vi "Set Switch Heater.vi"(1 "error in":T2, 2 "Switch Heater Control":bool, 3 "Communications Config":T1={"GPIB address"=22, "GPIB bus"=0, "connection ID"=refnum, "IP"="192.168.2.200", "Active Comm Interface"=0, "Serial Port"="", "Programmer Type"=0} {"Programmer Type" items=["Model 430", "Model 420"]; "Active Comm Interface" items=["TCP/IP (Model 430 Only)", "RS232", "IEEE488"]}) -> (0 "error out":T2)   [LabVIEW 2018]
panel:
  in  "GPIB Address":cluster{"GPIB address":i16, "GPIB bus":i16}={"GPIB address"=22, "GPIB bus"=0}
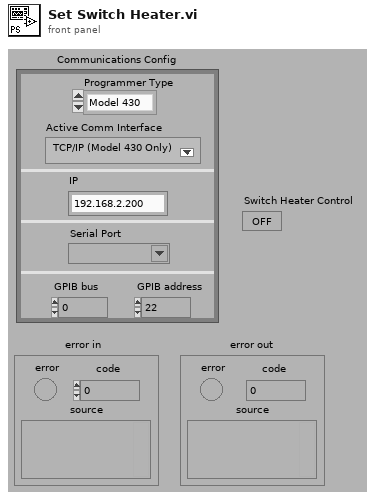
[diagram p1: front panel]
types:
  T1 = cluster{"GPIB address":i16, "GPIB bus":i16, "connection ID":refnum<k5>, "IP":string, "Active Comm Interface":u16, "Serial Port":refnum<visa-resource-name>, "Programmer Type":u16}
  T2 = cluster{"error":bool, "code":i32, "source":string}
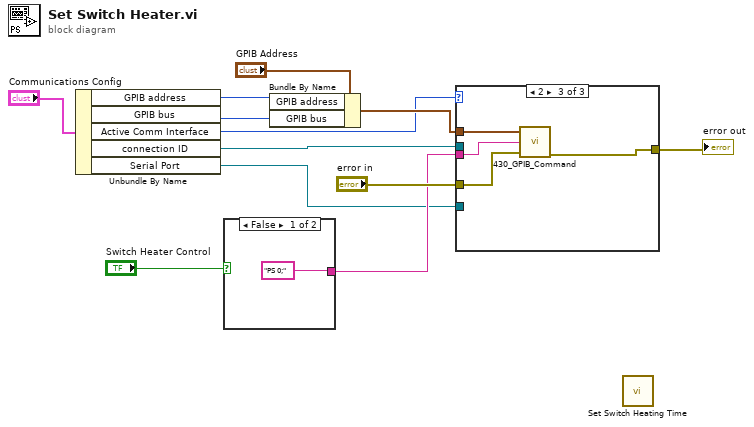
[diagram p0: block diagram]
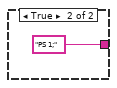
[diagram p2: hidden frame]
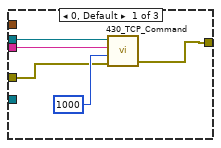
[diagram p3: hidden frame]
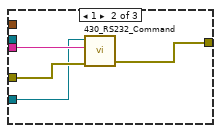
[diagram p4: hidden frame]
diagram:
  n1 = Unbundle By Name("Communications Config") -> ("GPIB address"=w6:i16, "GPIB bus"=w5:i16, "Active Comm Interface"=w4:u16, "connection ID"=w3:refnum<k5>, "Serial Port"=w2:refnum<visa-resource-name>)
  n2 = case shown="False" "Switch Heater Control" {
    tunnel: ["PS 0;" "PS 1;"] -> w8
    frame False {
    }
    frame True {
    }
  }
  n3 = Bundle By Name(cluster="GPIB Address", "GPIB address"=w6, "GPIB bus"=w5) -> (w7:cluster{"GPIB address":i16, "GPIB bus":i16})
  n4 = case shown="2" w4 {
    tunnel: w7 -> [_ _ w24]
    tunnel: "error in" -> [w18 w22 w27]
    tunnel: [w15 w21 w26] -> w11
    tunnel: w8 -> [w17 w23 w25]
    tunnel: w3 -> [w16 _ _]
    tunnel: w2 -> [_ w20 _]
    frame 0, Default {
      n5 = call "430_TCP_Command.vi"("error in (no error)"=w18, "Timeout"=1000, "Command"=w17, "connection ID"=w16) -> ("error out"=w15:errorcluster)  [unwired: 2 out]
    }
    frame 1 {
      n6 = call "430_RS232_Command.vi"("error in (no error)"=w22, "Command"=w23, "VISA resource name"=w20) -> ("error out"=w21:errorcluster)  [unwired: 1 in, 2 out]
    }
    frame 2 {
      n7 = call "430_GPIB_Command.vi"("GPIB (In)"=w24, "Input command"=w25, "error in"=w27) -> ("error out"=w26:T2)  [unwired: 3 out]
    }
  }
  "error out" <- w11
  n8 = call "Set Switch Heating Time.vi"() -> ()  [unwired: 3 in, 1 out]
